vi "Elevator Position Global.vi"() -> ()   [LabVIEW 2017]
panel:
  in  "Position Norm":dbl
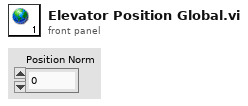
[diagram p1: front panel]
diagram:
